vi "random gen2.vi"() -> (0 "Init Data Out":i16[](array[numeric]))   [LabVIEW 2015]
panel:
  in  "Max":dbl=65534.0
  # "For Initialization VI requirements and help, please read directions located on Block Diagram."
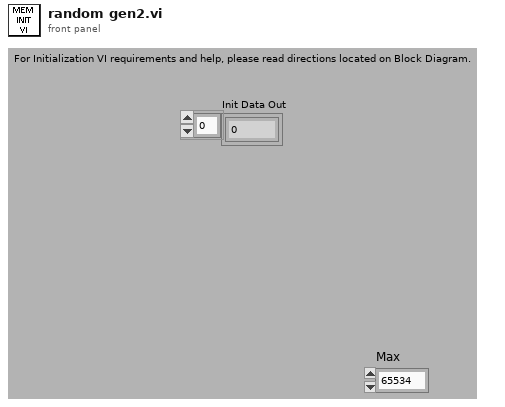
[diagram p1: front panel]
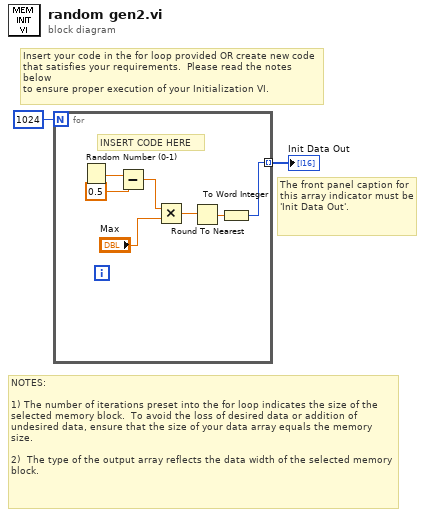
[diagram p0: block diagram]
diagram:
  # "The front panel caption for this array indicator must be 'Init Data Out'."
  # "NOTES:\n\n1) The number of iterations preset into the for loop indicates the size of the selected memory block.  To avoid the loss of desired data or addition of undesired data, ensure that the size of your data array equals the memory size.\n\n2)  The type of the output array reflects the data width of the selected memory block."
  # "Insert your code in the for loop provided OR create new code\nthat satisfies your requirements.  Please read the notes below\nto ensure proper execution of your Initialization VI."
  n1 = for {
    N: u32 1024 -> [_]
    tunnel: [w3] -> w1 mode=indexing
    # "INSERT CODE HERE"
    n2 = Random Number (0-1)() -> (number: 0 to 1=w6:dbl)
    n3 = Subtract(x=w6, y=0.5) -> (x-y=w7:dbl)
    n4 = Multiply(x=w7, y="Max") -> (x*y=w5:dbl)
    n5 = Round To Nearest(number=w5) -> (nearest integer value=w9:dbl)
    n6 = To Word Integer(number=w9) -> (16bit integer=w3:i16)
  }
  "Init Data Out" <- w1
